vi "ReadWriteTopicData.vi"(3 "error in (no error)":errorcluster, 4 "timeout ms (1000)":i32=1000, 5 "connection ID in":refnum<k5>) -> (0 "error out":errorcluster, 1 "data out":string, 2 "connection ID out":refnum<k5>)   [LabVIEW 2015]
uses:
  MessageParsing/std_msgs/subs/parse_u32_scalar.vi
panel:
  out "received":i32
  out "requested":u32
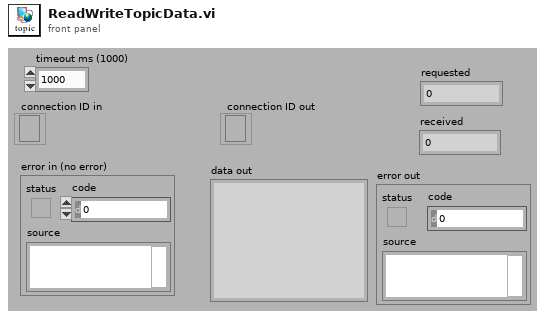
[diagram p1: front panel]
types:
  T1 = enum16{"Standard", "Buffered", "CRLF", "Immediate"}
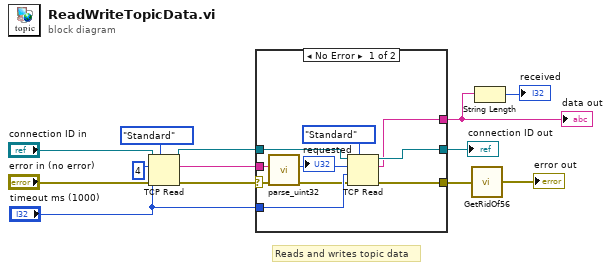
[diagram p0: block diagram]
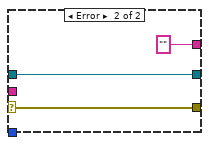
[diagram p2: hidden frame]
diagram:
  # "Reads and writes topic data"
  n1 = TCP Read(connection ID="connection ID in", bytes to read=4, error in (no error)="error in (no error)", 7:T1."Standard" ("mode (standard)"), 9:"timeout ms (1000)") -> (connection ID out=w11:refnum<k5>, data out=w8:string, error out=w7:errorcluster)
  n2 = case shown="No Error" w7 {
    selector: w7 -> [w15 w24]
    tunnel: [w14 "" ("data out")] -> w4
    tunnel: [w23 w24] -> w1
    tunnel: [w22 w26] -> w2
    tunnel: w11 -> [w21 w26]
    tunnel: w8 -> [w16 _]
    tunnel: "timeout ms (1000)" -> [w19 _]
    frame No Error {
      n3 = call-poly "parse_uint32.vi"("error in"=w15, "msg in"=w16) -> ("error out"=w17:errorcluster, "number"=w18:u32)  [unwired: 3 in, 1 out]
      "requested" <- w18
      n4 = TCP Read(connection ID=w21, bytes to read=w18, error in (no error)=w17, 7:T1."Standard" ("mode (standard)"), 9:w19) -> (connection ID out=w22:refnum<k5>, data out=w14:string, error out=w23:errorcluster)
    }
    frame Error {
    }
  }
  "data out" <- w4
  "connection ID out" <- w2
  n5 = call "GetRidOf56.vi"("error in (no error)"=w1) -> ("error out"=→"error out":errorcluster)
  n6 = String Length(string=w4) -> (length=→"received":i32)
